vi "Initalize.vi"(8 "error in (no error)":errorcluster, 9 "Section":string, 10 "Config Path":path, 11 "Dynamic Load in":refnum<class "Dynamic Load.lvclass">) -> (0 "error out":errorcluster, 3 "Dynamic Load out":refnum<class "Dynamic Load.lvclass">)   [LabVIEW 2022 SP3, in "Dynamic Load.lvclass"]
uses:
  Dynamic Load.lvclass
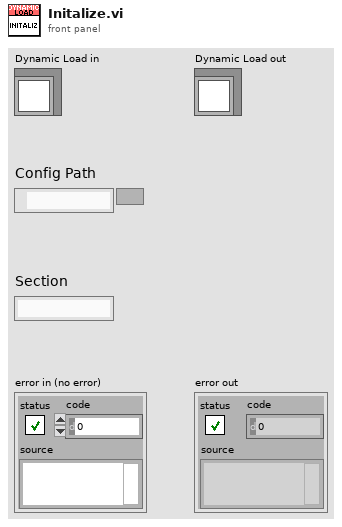
[diagram p1: front panel]
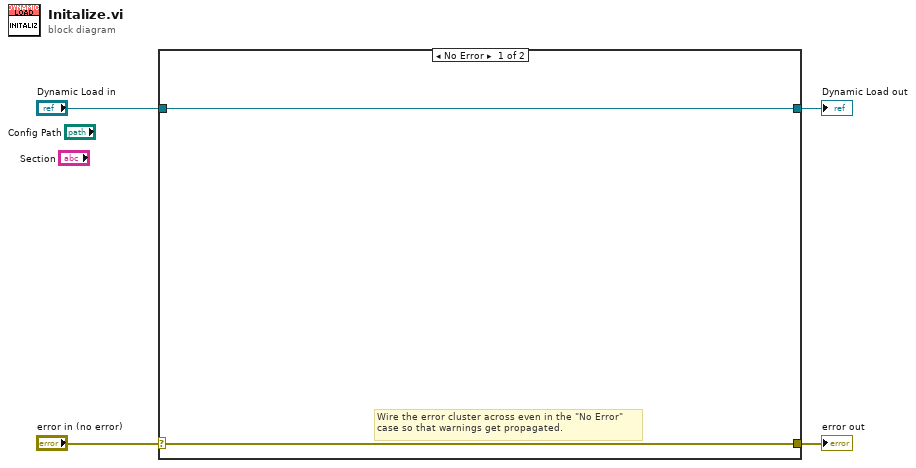
[diagram p0: block diagram]
diagram:
  n1 = case shown="No Error" "error in (no error)" {
    selector: "error in (no error)" -> [w5 w8]
    tunnel: [w5 w8] -> w3
    tunnel: [w6 w7] -> w1
    tunnel: "Dynamic Load in" -> [w6 w7]
    frame No Error {
      # "Wire the error cluster across even in the \"No Error\"\ncase so that warnings get propagated."
    }
    frame Error {
    }
  }
  "error out" <- w3
  "Dynamic Load out" <- w1
